vi "Ivium driver 1-03 - stripdown.vi"() -> ()   [LabVIEW 2020]
uses:
  Users/Benjamin/Desktop/StateMachine/Documents/LabVIEW Data/transmittance/controls/State.ctl
  IVIUM_remdriver.lvlib
panel:
  in  "cell potential":dbl caption="V" format="%_3p"
  out "cell on":bool
  out "current":dbl caption="A" format="%_4g"
  in  "Current range":T1(ring)=enum."10 mA"
  out "Device Status indicator":string
  out "cell-off button pressed":bool
  out "E_overload":bool
  out "Aninput1_overload":bool
  out "I_overload":bool
  in  "Set Filter":T2(ring)=enum."10 kHz"
  in  "Set Stability":T3(ring)=enum."Standard"
  in  "Tab Control Ac/external/bistat":enum32{"AC", "Extern", "BiStat"}(tab)
  in  "Record I":bool
  in  "Read and set values":bool
  in  "Exit and disconnect":bool
  out "Values to re-intialise to at end\nof the measument":T4
  out "Device serial number":string
  # "I overload"
  # "Cell-off button pressed"
  # "E overload"
  # "Aninput1 overload"
  # "Ac signal"
  # "Analog input"
  # "Digital output"
  # "Analog output"
  # "ch1"
  # "ch2"
  # "ch3"
  # "ch4"
  # "ch5"
  # "Digital input"
  # "ch6"
  # "ch7"
  # "ch8"
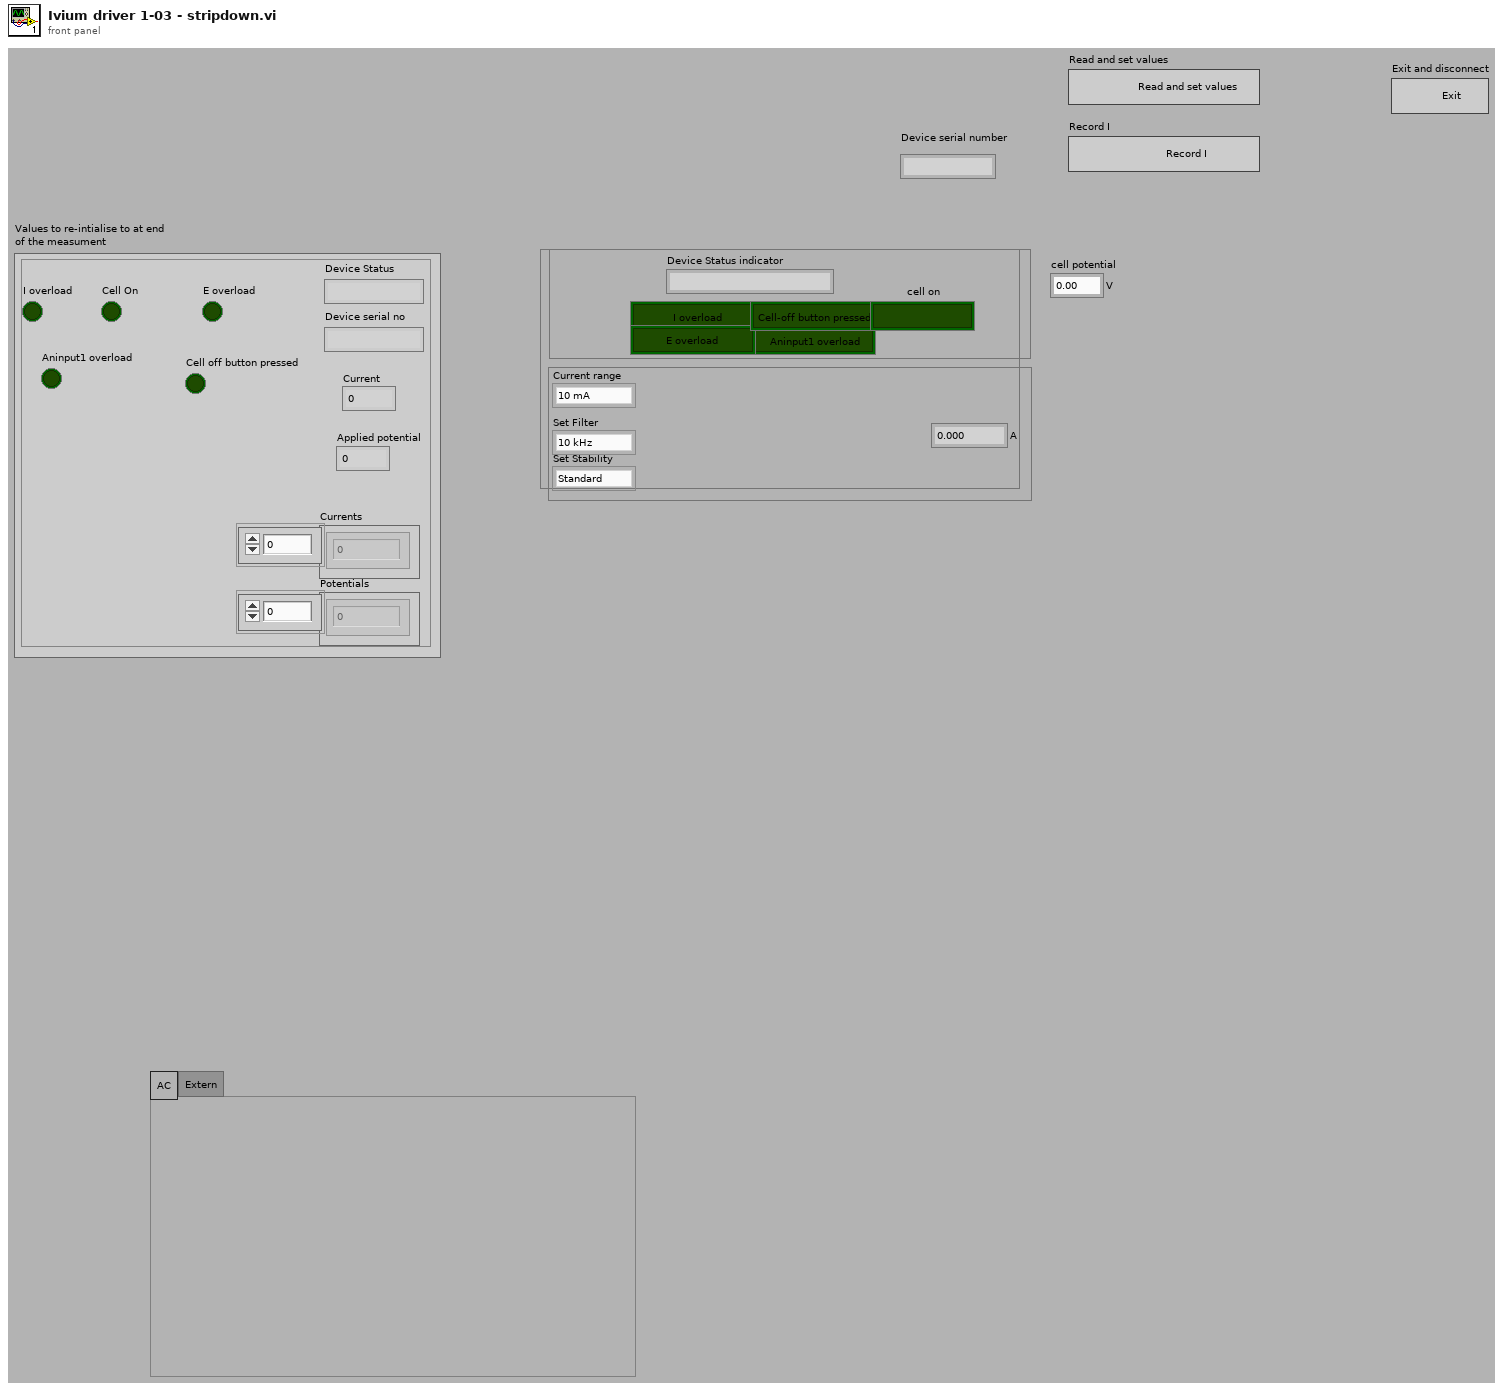
[diagram p1: front panel]
types:
  T1 = enum16{"10 A", "1 A", "100 mA", "10 mA", "1 mA", "100 uA", "10 uA", "1 uA", "100 nA", "10 nA", "1 nA", "100 pA", "10 pA", "1 pA"}
  T2 = enum16{"1 MHz", "100 kHz", "10 kHz", "1 kHz", "10 Hz"}
  T3 = enum16{"High Speed", "Standard", "High Stability"}
  T4 = cluster{"Currents":dbl[], "Potentials":dbl[], "Device Status":string, "Device serial no":string, "Current":dbl, "Applied potential":dbl, "I overload":bool, "Cell On":bool, "E overload":bool, "Aninput1 overload":bool, "Cell off button pressed":bool}
  T5 = cluster{"Current array":dbl[], "Potential array":dbl[], "Status":string, "Serial No":string, "Current":dbl, "Applied E":dbl, "I overload":bool, "Cell on":bool, "E overload":bool, "Cell of butt on pressed":bool, "Aninput1 overload":bool}
  T6 = typedef "State.ctl" = enum16{"Initialize", "Wait for Event", "Update and read", "Close ", "Output data and process", "Exit"}
  T7 = enum16{"off", "EStat4EL", "EStat2EL", "EStatDummy1", "EStatDummy2", "EStatDummy3", "EStatDummy4", "IStat4EL", "IStat2EL", "IStatDummy", "BiStat4EL", "BiStat2EL"}
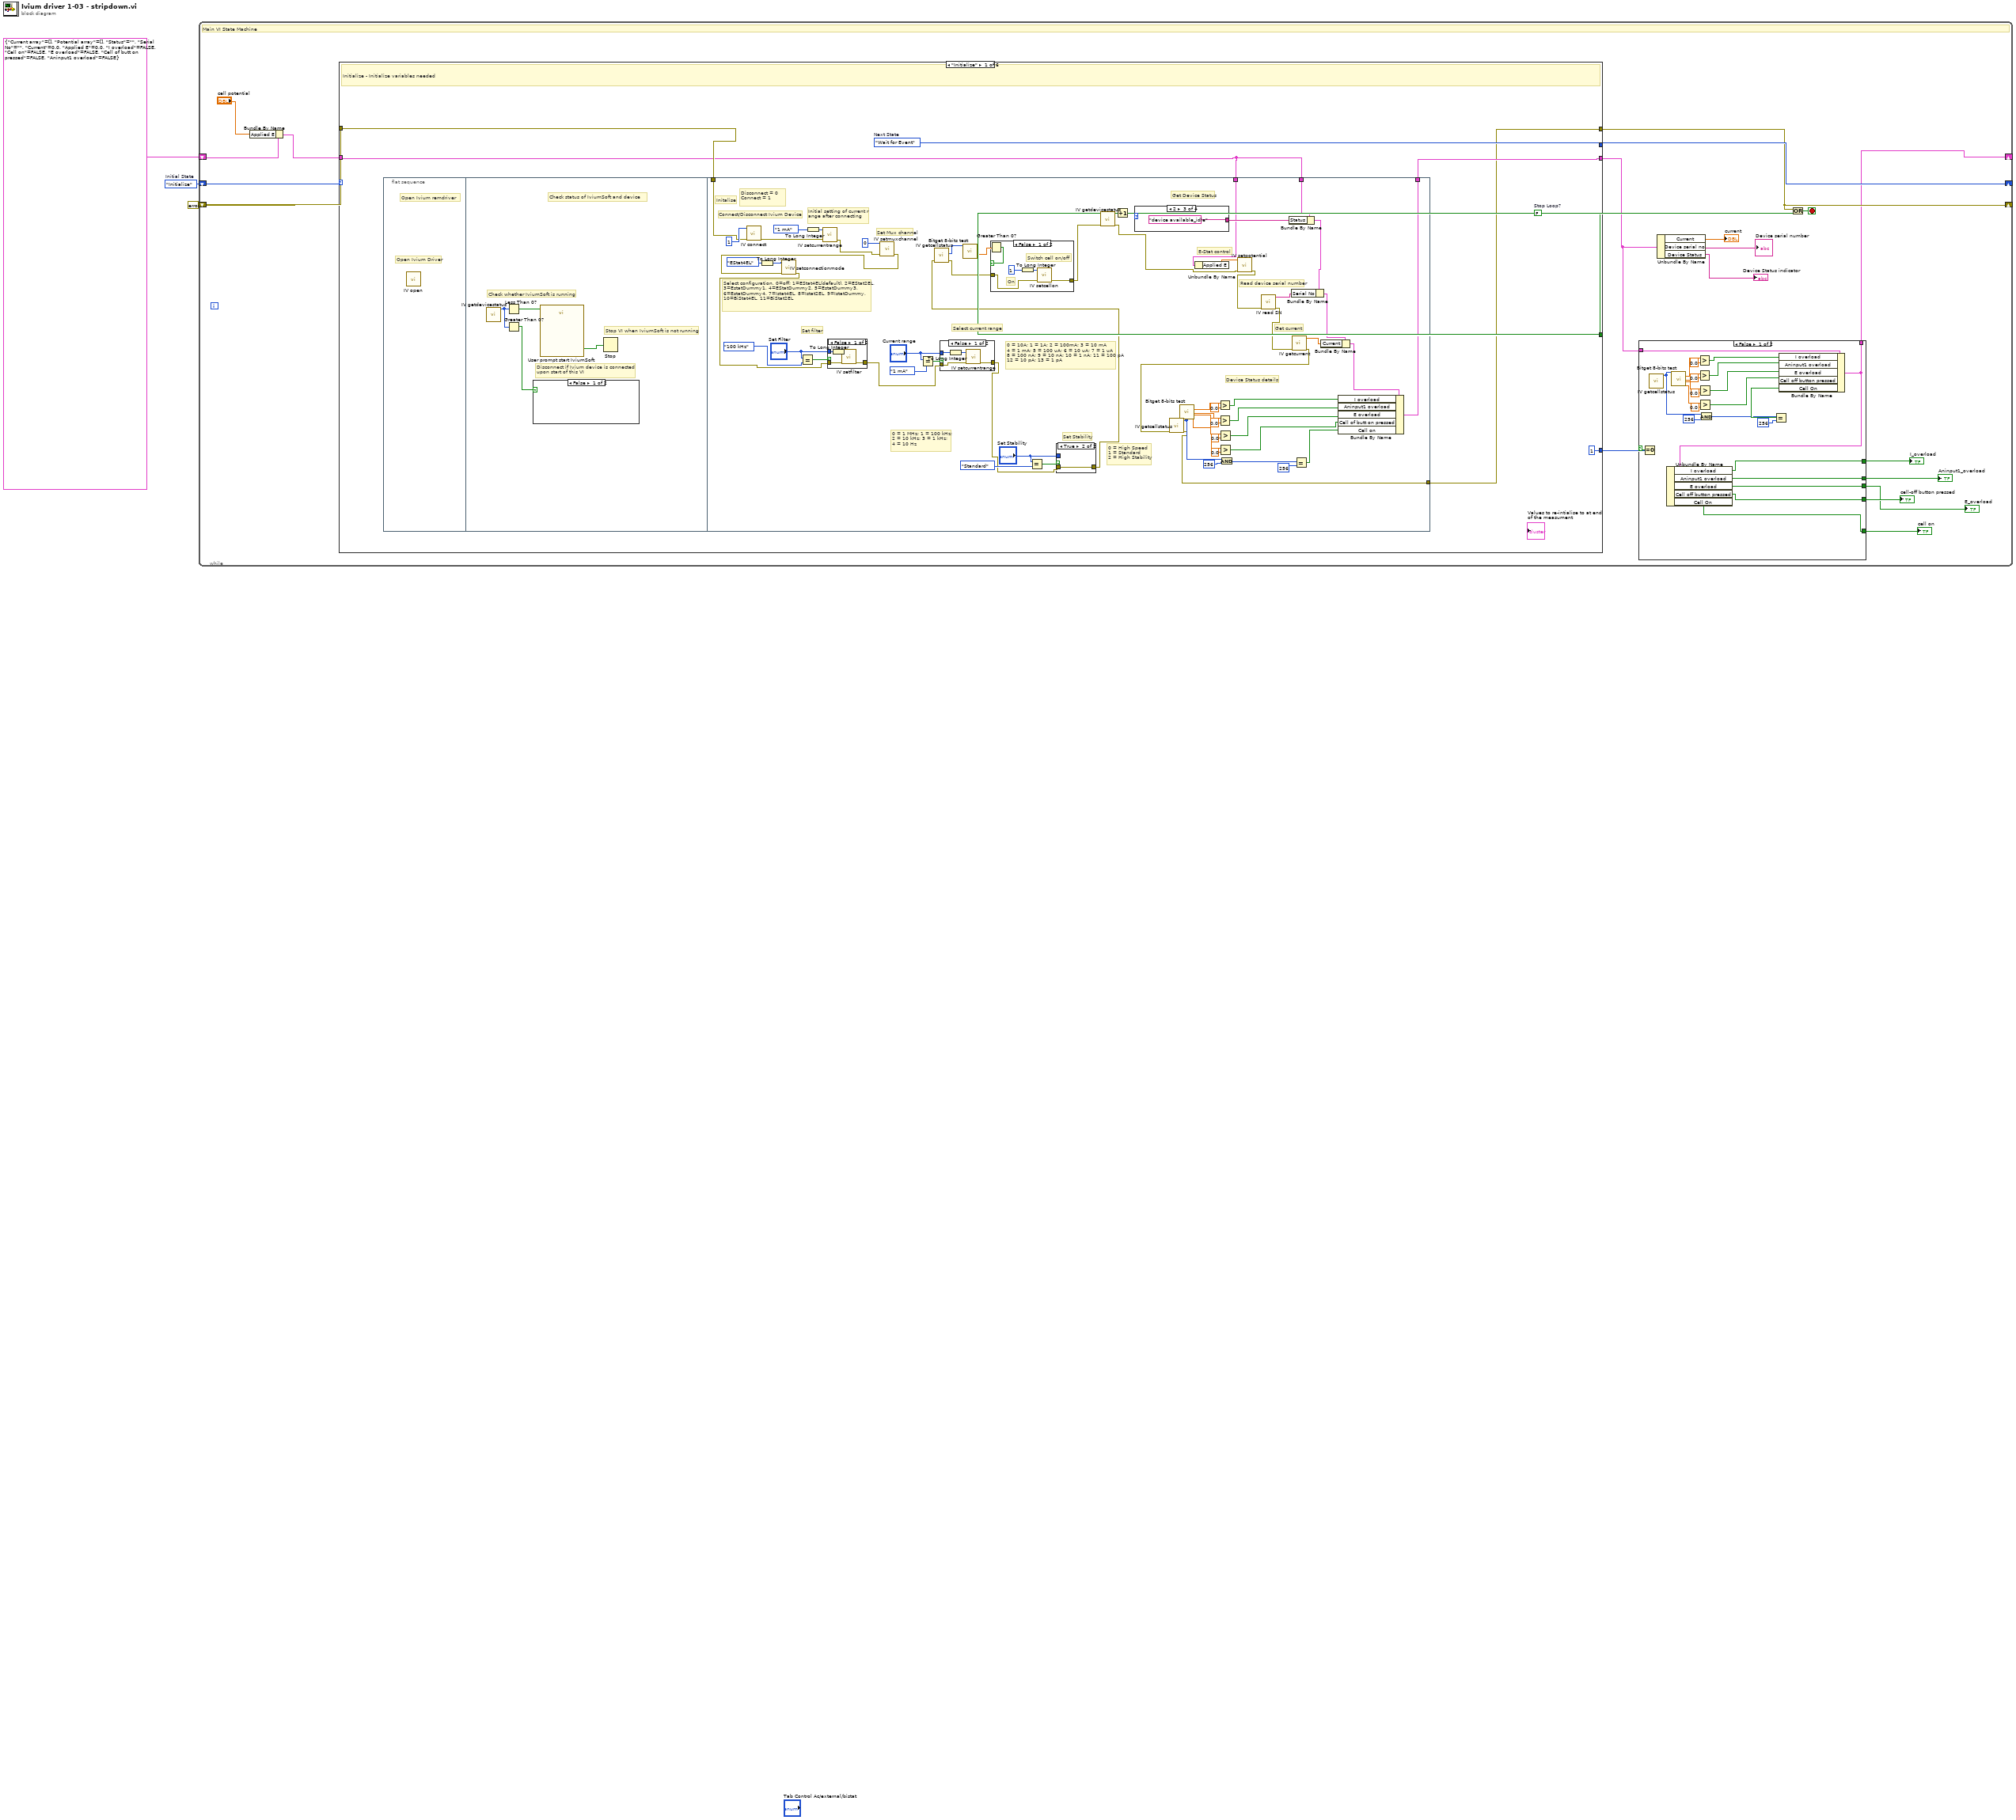
[diagram p0: block diagram]
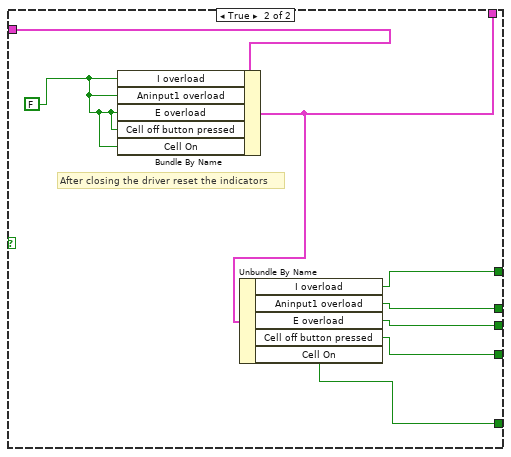
[diagram p2: hidden frame]
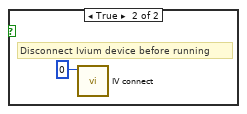
[diagram p3: hidden frame]
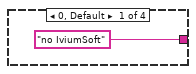
[diagram p5: hidden frame]
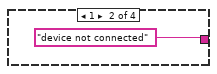
[diagram p6: hidden frame]
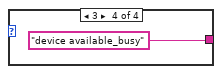
[diagram p7: hidden frame]
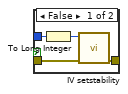
[diagram p8: hidden frame]
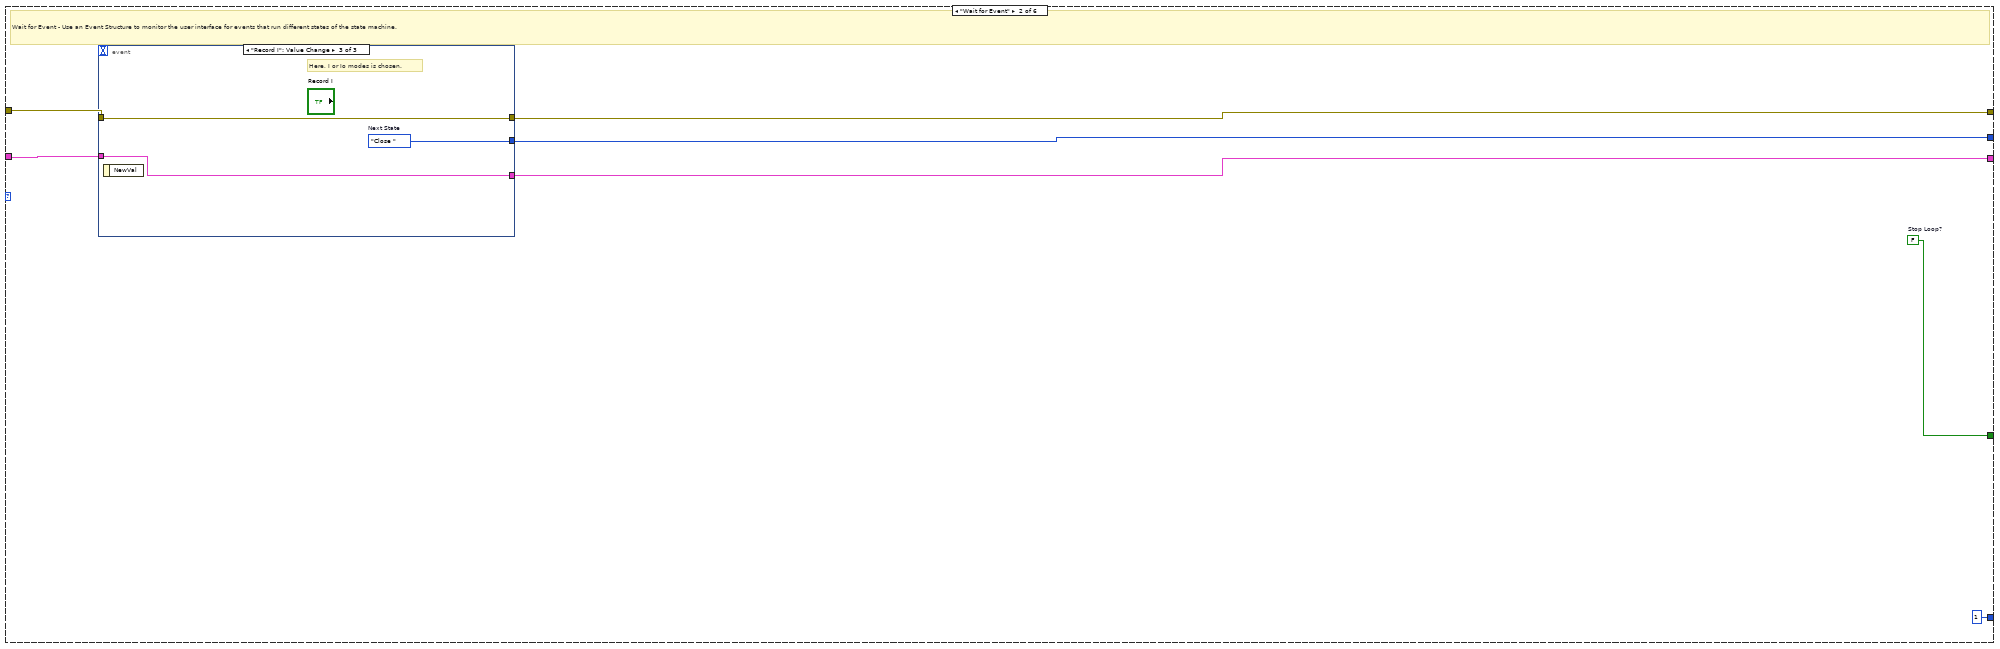
[diagram p11: hidden frame]
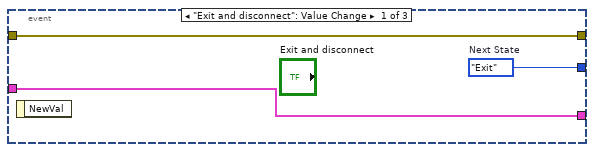
[diagram p12: hidden frame]
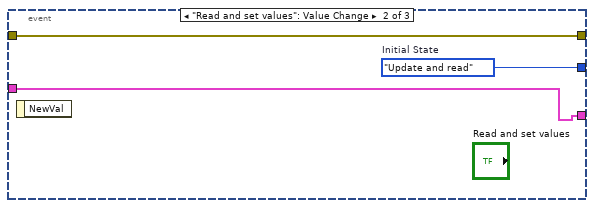
[diagram p13: hidden frame]
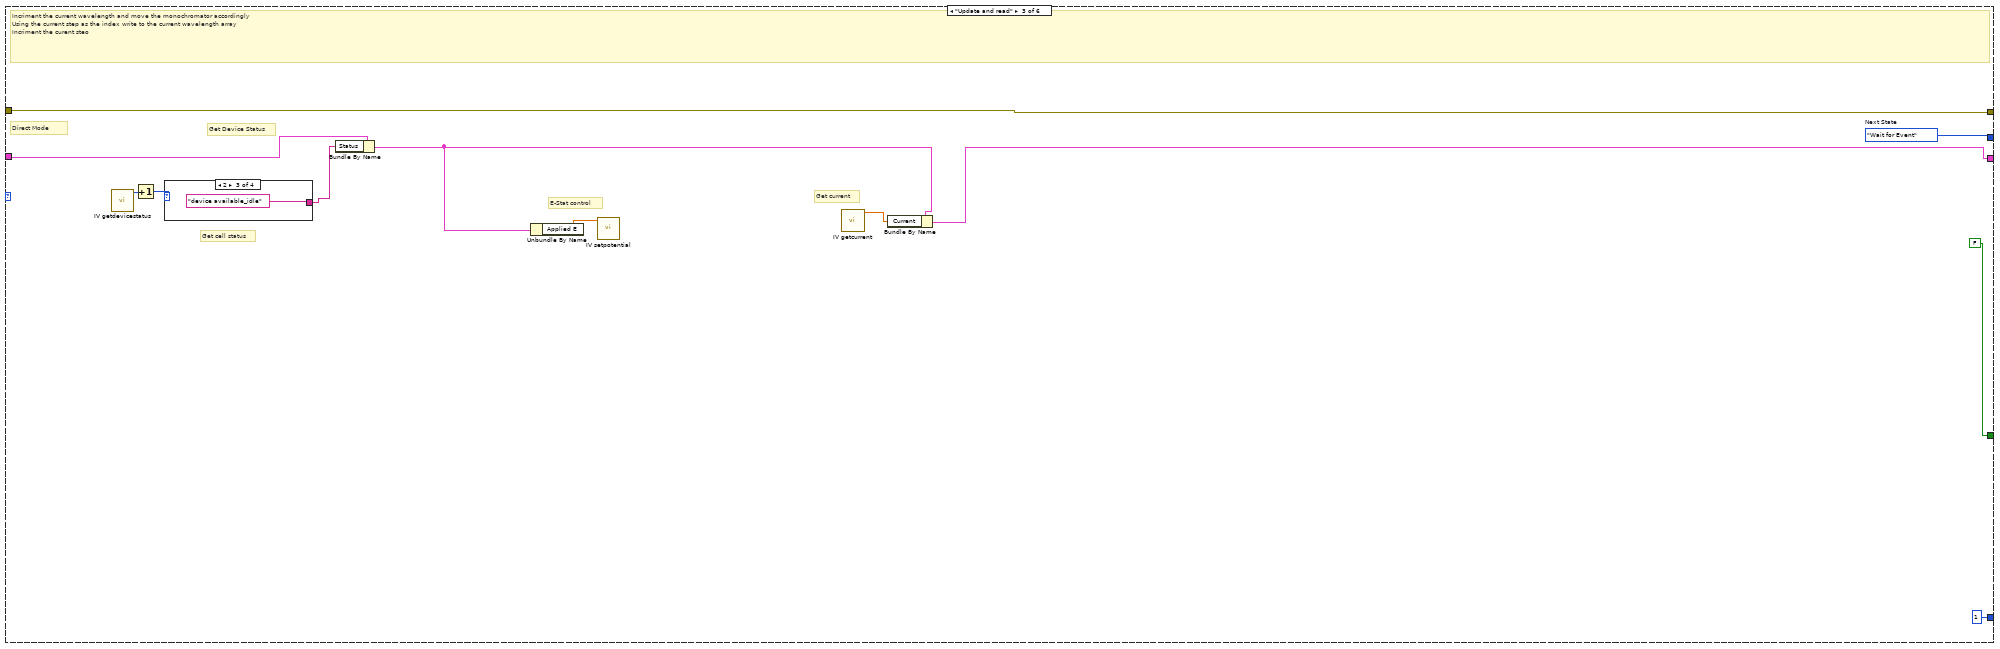
[diagram p14: hidden frame]
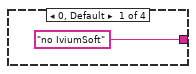
[diagram p15: hidden frame]
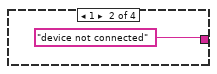
[diagram p16: hidden frame]
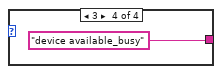
[diagram p17: hidden frame]
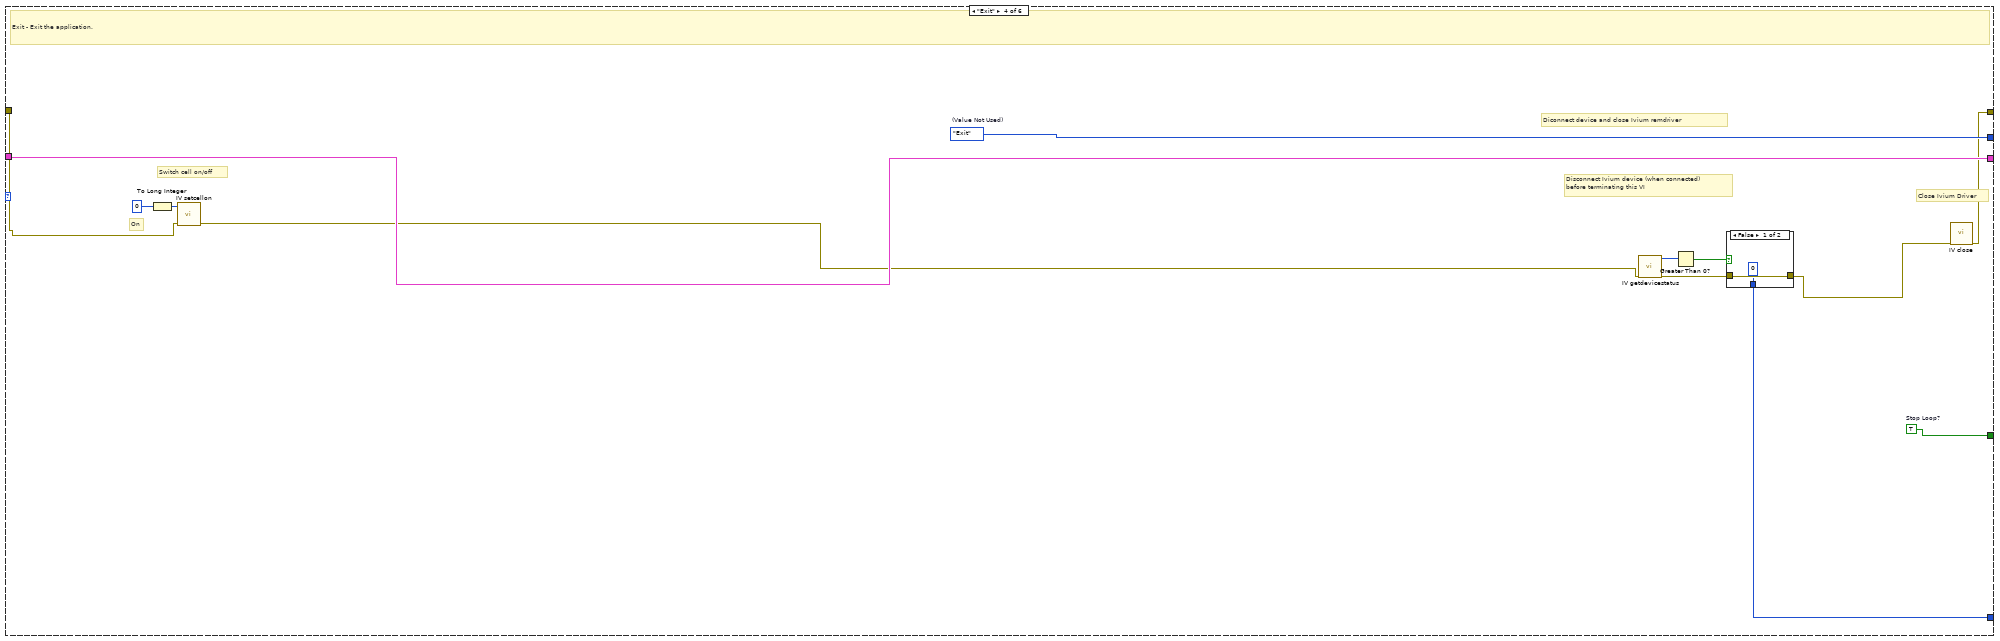
[diagram p18: hidden frame]
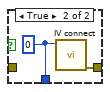
[diagram p19: hidden frame]
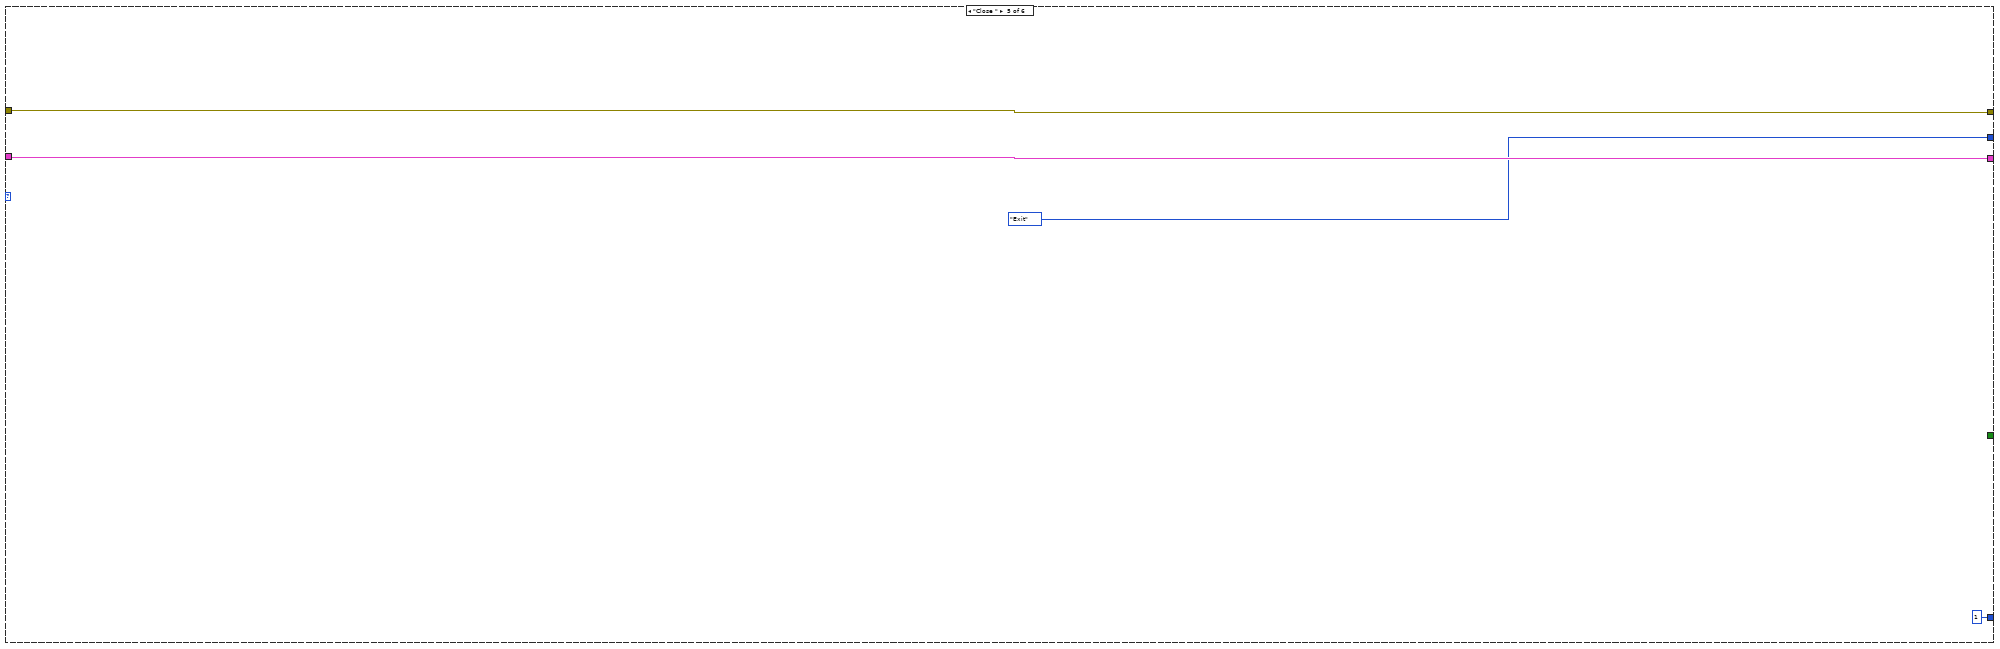
[diagram p20: hidden frame]
diagram:
  w3 = State."Initialize"  # Initial State
  n1 = while {
    shift-right: [w23] -> _
    shift-left: w3 -> [w24]
    shift-right: [w11] -> _
    shift-left: T5 {"Current array"=[], "Potential array"=[], "Status"="", "Serial No"="", "Current"=0.0, "Applied E"=0.0, "I overload"=FALSE, "Cell on"=FALSE, "E overload"=FALSE, "Cell of butt on pressed"=FALSE, "Aninput1 overload"=FALSE} -> [w15]
    shift-right: [w19] -> _
    shift-left: errorcluster {"status"=FALSE, "code"=0, "source"=""} ("error constant") -> [w22]
    stop <- w20 stop-if-true
    # "Main VI State Machine"
    n2 = Bundle By Name(cluster=w15, "Applied E"="cell potential") -> (w13:T5)
    n3 = case shown="\"Initialize\"" w24 {
      tunnel: [w63 w161 w179 w199 State."Exit" ("f") State."Wait for Event" ("f")] -> w23
      tunnel: [w62 w156 FALSE ("Stop Loop?") w192 _ _] -> w21
      tunnel: w13 -> [w58 w158 w178 w198 w207 _]
      tunnel: [w61 w157 w171 w198 w207 w209] -> w12
      tunnel: w22 -> [w59 w160 w182 w189 w206 w211]
      tunnel: [w57 w159 w182 w193 w206 w211] -> w19
      tunnel: [1 ("devconnect") 1 ("devconnect") 1 ("devconnect") w187 1 ("devconnect") 1 ("devconnect")] -> w10
      frame "Initialize" {
        w62 = FALSE  # Stop Loop?
        w63 = State."Wait for Event"  # Next State
        # "Initialize - Initialize variables needed"
        n4 = flat-sequence {
          tunnel: w58 -> [w104]
          tunnel: [w92] -> w61
          tunnel: w59 -> [w87]
          tunnel: w58 -> [w76]
          tunnel: [w72] -> w57
          frame #0 {
            # "Open Ivium Driver"
            # "Open Ivium remdriver"
            n5 = call "IV open.vi"() -> ()  [unwired: 10 in, 2 out]
          }
          frame #1 {
            # "Check status of IviumSoft and device"
            # "Stop VI when IviumSoft is not running"
            # "Disconnect if Ivium device is connected \nupon start of this VI"
            # "Check whether IviumSoft is running"
            n6 = call "IV getdevicestatus.vi"() -> ("return type"=w67:i32)  [unwired: 10 in, 1 out]
            n7 = Less Than 0?(x=w67) -> (x < 0?=w64:bool)
            n8 = Greater Than 0?(x=w67) -> (x > 0?=w66:bool)
            n9 = case shown="False" w66 {
              frame False {
              }
              frame True {
                # "Disconnect Ivium device before running"
                n10 = call "IV connect.vi"("devconnect"=0) -> ()  [unwired: 8 in, 3 out]
              }
            }
            n11 = call "User prompt start IviumSoft.vi"("Enable"=w64) -> ("OK"=w65:bool)  [unwired: 17 in, 1 out]
            n12 = Stop(stop? (T)=w65) -> ()
          }
          frame #2 {
            # "Device Status details"
            # "Get current"
            # "Set Mux channel"
            # "0 = High Speed\n1 = Standard \n2 = High Stability"
            # "Set Stability"
            # "0 = 1 MHz; 1 = 100 kHz; \n2 = 10 kHz; 3 = 1 kHz; \n4 = 10 Hz"
            # "Set filter"
            # "E-Stat control"
            # "Get Device Status"
            # "0 = 10A; 1 = 1A; 2 = 100mA; 3 = 10 mA\n4 = 1 mA; 5 = 100 uA; 6 = 10 uA; 7 = 1 uA\n8 = 100 nA; 9 = 10 nA; 10 = 1 nA; 11 = 100 pA\n12 = 10 pA; 13 = 1 pA"
            # "Select current range"
            # "Select configuration, 0=off; 1=EStat4EL(default), 2=EStat2EL, 3=EstatDummy1, 4=EStatDummy2, 5=EstatDummy3, 6=EstatDummy4, 7=Istat4EL, 8=Istat2EL, 9=IstatDummy, 10=BiStat4EL, 11=BiStat2EL"
            # "Read device serial number"
            # "Initial setting of current r\nange after connecting"
            # "Disconnect = 0\nConnect = 1"
            # "Connect/Disconnect Ivium Device"
            # "Initalise"
            n13 = call "IV connect.vi"("error in (no error)"=w87, "devconnect"=1) -> ("error out"=w84:errorcluster)  [unwired: 7 in, 2 out]
            n14 = To Long Integer(number=T7."EStat4EL" ("Configuration")) -> (32bit integer=w106:i32)
            n15 = Equal?(x="Set Filter", y=T2."100 kHz" ("Set Filter")) -> (x = y?=w124:bool)
            n16 = To Long Integer(number=T1."1 mA" ("Current range selector")) -> (32bit integer=w86:i32)
            n17 = call "IV setcurrentrange.vi"("error in (no error)"=w84, "value"=w86) -> ("error out"=w71:errorcluster)  [unwired: 7 in, 2 out]
            n18 = call "IV setmuxchannel.vi"("error in (no error)"=w71, "value"=0) -> ("error out"=w79:errorcluster)  [unwired: 7 in, 2 out]
            n19 = call "IV setconnectionmode.vi"("error in (no error)"=w79, "value"=w106) -> ("error out"=w83:errorcluster)  [unwired: 7 in, 2 out]
            n20 = case shown="False" w124 {
              tunnel: "Set Filter" -> [w148 _]
              tunnel: w83 -> [w146 w149]
              tunnel: [w145 w149] -> w82
              frame False {
                n21 = To Long Integer(number=w148) -> (32bit integer=w147:i32)
                n22 = call "IV setfilter.vi"("error in (no error)"=w146, "value"=w147) -> ("error out"=w145:errorcluster)  [unwired: 7 in, 2 out]
              }
              frame True {
              }
            }
            n23 = Equal?(x="Current range", y=T1."1 mA") -> (x = y?=w128:bool)
            n24 = case shown="False" w128 {
              tunnel: "Current range" -> [w152 _]
              tunnel: w82 -> [w151 w154]
              tunnel: [w150 w154] -> w78
              frame False {
                n25 = To Long Integer(number=w152) -> (32bit integer=w153:i32)
                n26 = call "IV setcurrentrange.vi"("error in (no error)"=w151, "value"=w153) -> ("error out"=w150:errorcluster)  [unwired: 7 in, 2 out]
              }
              frame True {
              }
            }
            n27 = Equal?(x="Set Stability", y=T3."Standard" ("Set Stability")) -> (x = y?=w126:bool)
            n28 = case shown="True" w126 {
              tunnel: "Set Stability" -> [w143 _]
              tunnel: w78 -> [w141 w144]
              tunnel: [w140 w144] -> w70
              frame False {
                n29 = To Long Integer(number=w143) -> (32bit integer=w142:i32)
                n30 = call "IV setstability.vi"("error in (no error)"=w141, "value"=w142) -> ("error out"=w140:errorcluster)  [unwired: 7 in, 2 out]
              }
              frame True {
              }
            }
            n31 = call "IV getcellstatus.vi"("error in (no error)"=w70) -> ("error out"=w81:errorcluster, "return type"=w91:i32)  [unwired: 8 in, 1 out]
            n32 = call "Bitget 8-bits test.vi"("x"=w91) -> ("f"=w90:dbl)  [unwired: 19 in, 7 out]
            n33 = Greater Than 0?(x=w90) -> (x > 0?=w89:bool)
            n34 = case shown="False" w89 {
              tunnel: w81 -> [w132 w135]
              tunnel: [w131 w135] -> w69
              frame False {
                # "On"
                # "Switch cell on/off"
                n35 = To Long Integer(number=1) -> (32bit integer=w134:i32)
                n36 = call "IV setcellon.vi"("error in (no error)"=w132, "cellon"=w134) -> ("error out"=w131:errorcluster)  [unwired: 7 in, 2 out]
              }
              frame True {
                # "If the cell is already\n on do nothing here"
              }
            }
            n37 = call "IV getdevicestatus.vi"("error in (no error)"=w69) -> ("error out"=w77:errorcluster, "return type"=w121:i32)  [unwired: 9 in]
            n38 = Increment(x=w121) -> (x+1=w120:i32)
            n39 = case shown="2" w120 {
              tunnel: ["no IviumSoft" "device not connected" "device available_idle" "device available_busy"] -> w105
              frame 0, Default {
              }
              frame 1 {
              }
              frame 2 {
              }
              frame 3 {
              }
            }
            n40 = Unbundle By Name(w76) -> ("Applied E"=w99:dbl)
            n41 = call "IV setpotential.vi"("error in (no error)"=w77, "value"=w99) -> ("error out"=w75:errorcluster)  [unwired: 7 in, 2 out]
            n42 = call "IV read SN.vi"("error in (no error)"=w75) -> ("error out"=w74:errorcluster, "sntext out"=w103:string)  [unwired: 8 in, 1 out]
            n43 = Bundle By Name(cluster=w104, "Status"=w105) -> (w102:T5)
            n44 = Bundle By Name(cluster=w102, "Serial No"=w103) -> (w101:T5)
            n45 = call "IV getcurrent.vi"("error in (no error)"=w74) -> ("error out"=w73:errorcluster, "value out"=w100:dbl)  [unwired: 8 in, 1 out]
            n46 = call "IV getcellstatus.vi"("error in (no error)"=w73) -> ("error out"=w72:errorcluster, "devcellstatus out"=w111:i32)  [unwired: 8 in, 1 out]
            n47 = call "Bitget 8-bits test.vi"("x"=w111) -> ("c"=w115:dbl, "e"=w113:dbl, "f"=w114:dbl, "h"=w112:dbl)  [unwired: 19 in, 4 out]
            n48 = Greater?(x=w115, y=0.0) -> (0:w97:bool)
            n49 = Greater?(x=w113, y=0.0) -> (0:w96:bool)
            n50 = Greater?(x=w114, y=0.0) -> (0:w95:bool)
            n51 = Greater?(x=w112, y=0.0) -> (0:w94:bool)
            n52 = And(x=w111, y=256) -> (x .and. y?=w109:i32)
            n53 = Equal?(x=w109, y=256) -> (x = y?=w93:bool)
            n54 = Bundle By Name(cluster=w101, "Current"=w100) -> (w98:T5)
            n55 = Bundle By Name(cluster=w98, "I overload"=w97, "Aninput1 overload"=w96, "E overload"=w95, "Cell of butt on pressed"=w94, "Cell on"=w93) -> (w92:T5)
          }
        }
      }
      frame "Wait for Event" {
        w156 = FALSE  # Stop Loop?
        # "Wait for Event - Use an Event Structure to monitor the user interface for events that run different states of the state machine."
        n56 = event shown="[2] \"Record I\": Value Change" {
          selector: _ -> [_ _ _]
          dyn-events: _ -> [_ _ _]
          timeout: _ -> [_ _ _]
          tunnel: [w164 w166 w170] -> w161
          tunnel: [w162 w165 w168] -> w157
          tunnel: w160 -> [w163 w167 w169]
          tunnel: [w163 w167 w169] -> w159
          tunnel: w158 -> [w162 w165 w168]
          event "Exit and disconnect": Value Change {
            w164 = State."Exit"  # Next State
            n57 = event-data() -> ()  [unwired: 1 in, 1 out]
          }
          event "Read and set values": Value Change {
            w166 = State."Update and read"  # Initial State
            n58 = event-data() -> ()  [unwired: 1 in, 1 out]
          }
          event "Record I": Value Change {
            w170 = State."Close "  # Next State
            # "Here, I or Io modes is chosen."
            n59 = event-data() -> ()  [unwired: 1 in, 1 out]
          }
        }
      }
      frame "Update and read" {
        w179 = State."Wait for Event"  # Next State
        # "Get current"
        # "E-Stat control"
        # "Get cell status"
        # "Get Device Status"
        # "Direct Mode"
        # "Incriment the current wavelength and move the monochromator accordingly\nUsing the current step as the index write to the current wavelength array\nIncriment the curent steo"
        n60 = call "IV getdevicestatus.vi"() -> ("return type"=w176:i32)  [unwired: 10 in, 1 out]
        n61 = Increment(x=w176) -> (x+1=w175:i32)
        n62 = case shown="2" w175 {
          tunnel: ["no IviumSoft" "device not connected" "device available_idle" "device available_busy"] -> w181
          frame 0, Default {
          }
          frame 1 {
          }
          frame 2 {
          }
          frame 3 {
          }
        }
        n63 = Bundle By Name(cluster=w178, "Status"=w181) -> (w172:T5)
        n64 = Unbundle By Name(w172) -> ("Applied E"=w174:dbl)
        n65 = call "IV setpotential.vi"("value"=w174) -> ()  [unwired: 8 in, 3 out]
        n66 = call "IV getcurrent.vi"() -> ("value out"=w173:dbl)  [unwired: 9 in, 2 out]
        n67 = Bundle By Name(cluster=w172, "Current"=w173) -> (w171:T5)
      }
      frame "Exit" {
        w192 = TRUE  # Stop Loop?
        w199 = State."Exit"  # (Value Not Used)
        # "On"
        # "Switch cell on/off"
        # "Diconnect device and close Ivium remdriver"
        # "Disconnect Ivium device (when connected)\nbefore terminating this VI"
        # "Close Ivium Driver"
        # "Exit - Exit the application."
        n68 = To Long Integer(number=0) -> (32bit integer=w191:i32)
        n69 = call "IV setcellon.vi"("error in (no error)"=w189, "cellon"=w191) -> ("error out"=w188:errorcluster)  [unwired: 7 in, 2 out]
        n70 = call "IV getdevicestatus.vi"("error in (no error)"=w188) -> ("error out"=w194:errorcluster, "return type"=w196:i32)  [unwired: 9 in]
        n71 = Greater Than 0?(x=w196) -> (x > 0?=w195:bool)
        n72 = case shown="False" w195 {
          tunnel: [w201 w203] -> w197
          tunnel: w194 -> [w201 _]
          tunnel: [0 ("devconnect") w202] -> w187
          frame False {
          }
          frame True {
            w202 = 0 ("devconnect")
            n73 = call "IV connect.vi"("devconnect"=w202) -> ("error out"=w203:errorcluster)  [unwired: 8 in, 2 out]
          }
        }
        n74 = call "IV close.vi"("error in (no error)"=w197) -> ("error out"=w193:errorcluster)  [unwired: 9 in, 1 out]
      }
      frame "Close " {
      }
      frame "Output data and process" {
        # "Also re-intialise constants"
        n75 = local read "Values to re-intialise to at end\nof the measument"() -> (w209:T4)
      }
    }
    n76 = Equal To 0?(x=w10) -> (x = 0?=w9:bool)
    n77 = case shown="False" w9 {
      tunnel: w12 -> [w33 w56]
      tunnel: [w31 w50] -> w11
      tunnel: [w29 w51] -> w8
      tunnel: [w28 w52] -> w7
      tunnel: [w27 w53] -> w6
      tunnel: [w26 w54] -> w5
      tunnel: [w25 w49] -> w4
      frame False {
        n78 = call "IV getcellstatus.vi"() -> ("devcellstatus out"=w43:i32)  [unwired: 9 in, 2 out]
        n79 = call "Bitget 8-bits test.vi"("x"=w43) -> ("c"=w39:dbl, "e"=w41:dbl, "f"=w40:dbl, "h"=w42:dbl)  [unwired: 19 in, 4 out]
        n80 = Greater?(x=w39, y=0.0) -> (0:w45:bool)
        n81 = Greater?(x=w41, y=0.0) -> (0:w46:bool)
        n82 = Greater?(x=w40, y=0.0) -> (0:w47:bool)
        n83 = Greater?(x=w42, y=0.0) -> (0:w32:bool)
        n84 = And(x=w43, y=256) -> (x .and. y?=w44:i32)
        n85 = Equal?(x=w44, y=256) -> (x = y?=w48:bool)
        n86 = Bundle By Name(cluster=w33, "I overload"=w45, "Aninput1 overload"=w46, "E overload"=w47, "Cell off button pressed"=w32, "Cell On"=w48) -> (w31:T4)
        n87 = Unbundle By Name(w31) -> ("I overload"=w26:bool, "Aninput1 overload"=w27:bool, "E overload"=w28:bool, "Cell off button pressed"=w29:bool, "Cell On"=w25:bool)
      }
      frame True {
        w55 = FALSE
        # "After closing the driver reset the indicators"
        n88 = Bundle By Name(cluster=w56, "I overload"=w55, "Aninput1 overload"=w55, "E overload"=w55, "Cell off button pressed"=w55, "Cell On"=w55) -> (w50:T4)
        n89 = Unbundle By Name(w50) -> ("I overload"=w54:bool, "Aninput1 overload"=w53:bool, "E overload"=w52:bool, "Cell off button pressed"=w51:bool, "Cell On"=w49:bool)
      }
    }
    "I_overload" <- w5
    "Aninput1_overload" <- w6
    "E_overload" <- w7
    "cell-off button pressed" <- w8
    "cell on" <- w4
    n90 = Unbundle By Name(w12) -> ("Current"=→"current":dbl, "Device serial no"=→"Device serial number":string, "Device Status"=→"Device Status indicator":string)
    n91 = Or(x=w19, y=w21) -> (x .or. y?=w20:bool)
  }
